vi "Recognize Goal.vi"(5 "Camera Type":T1=enum."MS HD3000 square", 6 "HSV":T5, 7 "Min Score Threshold":i32=70, 8 "Image Dst":T4, 9 "Image In":T4) -> (0 "Highest Average Score":dbl, 1 "Target With Highest Average Score":T2, 2 "All Targets Found":T3(array[cluster]) {"Normalized Rect"."Numeric 5" format="%#_2g"; "Normalized Rect"."Numeric 3" format="%#_2g"; "Normalized Rect"."Numeric 2" format="%#_2g"; "Normalized Rect"."Numeric" format="%#_2g"})   [LabVIEW 2015]
doc: "Performs target recognition on the image passed in. Returns all targets found. Each target includes distance in feet, center X/Y coordinates, and bounding rect coordinates (all coordinates are norminalized from -1 to 1). Also separately returns the target with the highest average score (i.e. most likely to be a real target)."
uses:
  <vilib>/vision/Image Controls.llb/IMAQ Image.ctl
  Camera Types.ctl
  <vilib>/vision/NI_Vision_Development_Module.lvlib
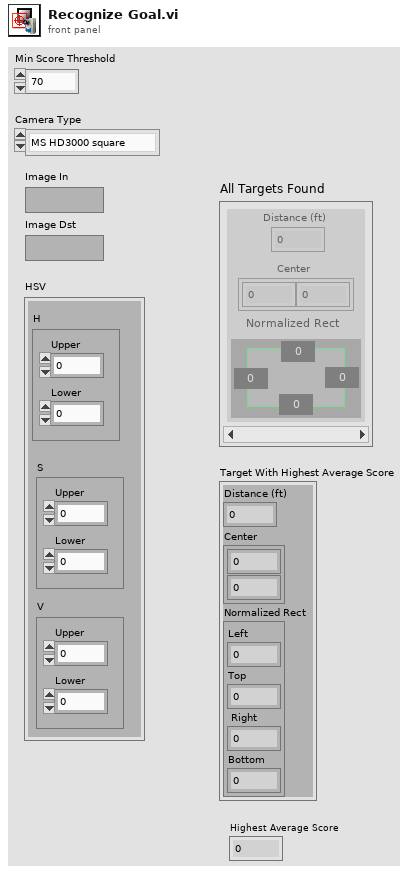
[diagram p1: front panel]
types:
  T1 = typedef "Camera Types.ctl" = enum16{"206", "1011", "1013", "MS HD3000 square", "MS HD3000 640x480"}
  T2 = cluster{"Distance (ft)":dbl, "Center":cluster{dbl, dbl}, "Normalized Rect":cluster{"Left":dbl, "Top":dbl, " Right":dbl, "Bottom":dbl}}
  T3 = cluster{"Distance (ft)":dbl, "Center":cluster{dbl, dbl}, "Normalized Rect":cluster{"Numeric":dbl, "Numeric 2":dbl, "Numeric 3":dbl, "Numeric 5":dbl}}[]
  T4 = typedef "IMAQ Image.ctl" = refnum<image>
  T5 = cluster{"H":cluster{"Upper":dbl, "Lower":dbl}, "S":cluster{"Upper":dbl, "Lower":dbl}, "V":cluster{"Upper":dbl, "Lower":dbl}}
  T6 = typedef "Particle Parameters" = i32
  T7 = cluster{"Bounding box":cluster{"left":dbl, "top":dbl, "right":dbl, "bottom":dbl}, "Aspect Ratio":dbl, "Area to CH":dbl, "X Mask":dbl, "Y Mask":dbl, "Moment":dbl}[]
  T8 = cluster{"Distance (ft)":dbl, "Center":cluster{dbl, dbl}, "Normalized Rect":cluster{"Numeric":dbl, "Numeric 2":dbl, "Numeric 3":dbl, "Numeric 5":dbl}}
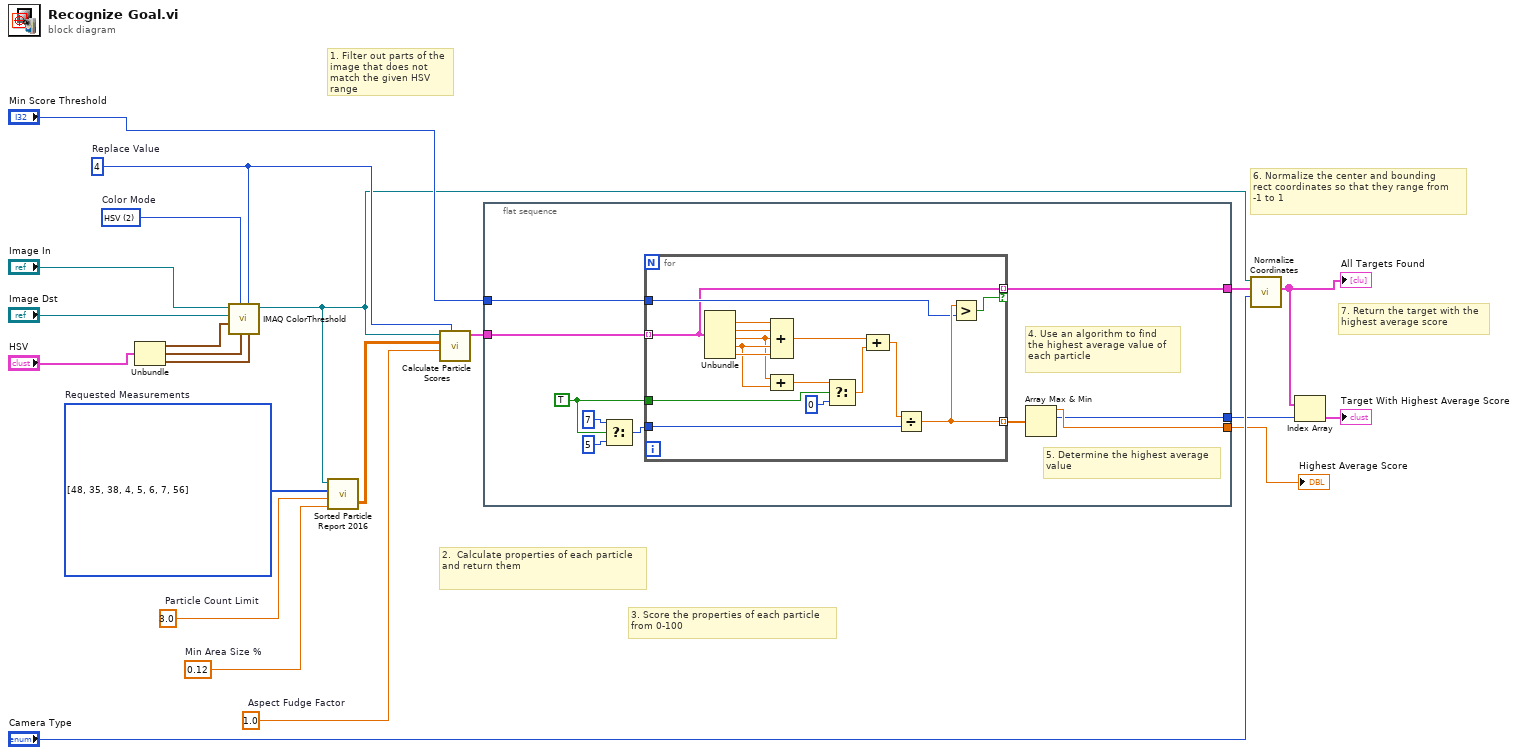
[diagram p0: block diagram]
diagram:
  w11 = 1.0  # Aspect Fudge Factor
  w12 = T6[] [48, 35, 38, 4, 5, 6, 7, 56] items=["Center of Mass X", "Center of Mass Y", "First Pixel X", "First Pixel Y", "Bounding Rect Left", "Bounding Rect Top", "Bounding Rect Right", "Bounding Rect Bottom", "Max Feret Diameter Start X", "Max Feret Diameter Start Y", "Max Feret Diameter End X", "Max Feret Diameter End Y", "Max Horiz. Segment Length Left", "Max Horiz. Segment Length Right", "Max Horiz. Segment Length Row", "-", "Bounding Rect Width", "Bounding Rect Height", "Bounding Rect Diagonal", "Perimeter", "Convex Hull Perimeter", "Holes' Perimeter", "Max Feret Diameter", "Equivalent Ellipse Major Axis", "Equivalent Ellipse Minor Axis", "Equivalent Ellipse Minor Axis (Feret)", "Equivalent Rect Long Side", "Equivalent Rect Short Side", "Equivalent Rect Diagonal", "Equivalent Rect Short Side (Feret)", "Average Horiz. Segment Length", "Average Vert. Segment Length", "Hydraulic Radius", "Waddel Disk Diameter", "-", "Area", "Holes' Area", "Particle & Holes' Area", "Convex Hull Area", "Image Area", "-", "Number of Holes", "Number of Horiz. Segments", "Number of Vert. Segments", "-", "Orientation", "Max Feret Diameter Orientation", "-", "% Area/Image Area", "% Area/(Particle & Holes' Area)", "Ratio of Equivalent Ellipse Axes", "Ratio of Equivalent Rect Sides", "-", "Elongation Factor", "Compactness Factor", "Heywood Circularity Factor", "Type Factor", "-", "Sum X", "Sum Y", "Sum XX", "Sum XY", "Sum YY", "Sum XXX", "Sum XXY", "Sum XYY", "Sum YYY", "-", "Moment of Inertia XX", "Moment of Inertia XY", "Moment of Inertia YY", "Moment of Inertia XXX", "Moment of Inertia XXY", "Moment of Inertia XYY", "Moment of Inertia YYY", "Norm. Moment of Inertia XX", "Norm. Moment of Inertia XY", "Norm. Moment of Inertia YY", "Norm. Moment of Inertia XXX", "Norm. Moment of Inertia XXY", "Norm. Moment of Inertia XYY", "Norm. Moment of Inertia YYY", "Hu Moment 1", "Hu Moment 2", "Hu Moment 3", "Hu Moment 4", "Hu Moment 5", "Hu Moment 6", "Hu Moment 7"]  # Requested Measurements
  w14 = 3.0  # Particle Count Limit
  w15 = 0.12  # Min Area Size %
  w8 = 4  # Replace Value
  w16 = u16 2 items=["RGB", "HSL", "HSV", "HSI"]  # Color Mode
  # "6. Normalize the center and bounding \nrect coordinates so that they range from\n-1 to 1"
  # "7. Return the target with the\nhighest average score"
  # "3. Score the properties of each particle \nfrom 0-100"
  # "2.  Calculate properties of each particle and return them"
  # "1. Filter out parts of the image that does not match the given HSV range"
  n1 = Unbundle("HSV") -> ("H"=w19:cluster{"Upper":dbl, "Lower":dbl}, "S"=w18:cluster{"Upper":dbl, "Lower":dbl}, "V"=w17:cluster{"Upper":dbl, "Lower":dbl})
  n2 = call "IMAQ ColorThreshold"("Blue or Luma or Val or Inten Range"=w17, "Replace Value"=w8, "Green or Sat Range"=w18, "Color Mode"=w16, "Red or Hue Range"=w19, "Image Dst"="Image Dst", "Image Src"="Image In") -> ("Image Dst Out"=w4:T4)  [unwired: 3 in, 1 out]
  n3 = call "Sorted Particle Report 2016.vi"("Min Area Size %"=w15, "Particle Count Limit"=w14, "Pixel Measurements"=w12, "Image in"=w4) -> ("Sorted Data"=w13:dbl[][])  [unwired: 1 out]
  n4 = call "Calculate Particle Scores.vi"("Pixel Value"=w8, "Aspect Fudge Factor"=w11, "Sorted Data"=w13, "Image in"=w4) -> ("Scores"=w10:T7)  [unwired: 7 in]
  n5 = flat-sequence {
    tunnel: w10 -> [w32]
    tunnel: "Min Score Threshold" -> [w31]
    tunnel: [w25] -> w5
    tunnel: [w24] -> w2
    tunnel: [w23] -> w1
    frame #0 {
      w27 = TRUE ("Emphasize Limit Tests")
      # "5. Determine the highest average\nvalue"
      # "4. Use an algorithm to find\nthe highest average value of \neach particle"
      n6 = Select(t=7, s=w27, f=5) -> (s? t:f=w28:i32)
      n7 = for {
        tunnel: w32 -> [w33] mode=indexing
        tunnel: [w33] -> w25 mode=indexing if=w46
        tunnel: [w45] -> w26 mode=indexing
        tunnel: w31 -> [w44]
        tunnel: w27 -> [w37]
        tunnel: w28 -> [w34]
        n8 = Unbundle(w33) -> ("Aspect Ratio"=w48:dbl, "Area to CH"=w47:dbl, "X Mask"=w39:dbl, "Y Mask"=w40:dbl, "Moment"=w41:dbl)  [unwired: 1 out]
        n9 = Compound Arithmetic op=ADD(w48, w47, w39, w40, w41) -> (w43:dbl)
        n10 = Compound Arithmetic op=ADD(w39, w40) -> (w38:dbl)
        n11 = Select(t=w38, s=w37, f=0) -> (s? t:f=w36:dbl)
        n12 = Compound Arithmetic op=ADD(w43, w36) -> (w42:dbl)
        n13 = Divide(x=w42, y=w34) -> (x/y=w45:dbl)
        n14 = Greater?(x=w45, y=w44) -> (0:w46:bool)
      }
      n15 = Array Max & Min(array=w26) -> (max value=w24:dbl, max index (indices)=w23:i32)  [unwired: 2 out]
    }
  }
  n16 = call "Normalize Coordinates.vi"("Camera Type"="Camera Type", "Targets"=w5, "Image in"=w4) -> ("Found Targets"=w7:T3)  [unwired: 7 in, 1 out]
  "All Targets Found" <- w7
  n17 = Index Array(array=w7, index=w1) -> (element=→"Target With Highest Average Score":T8)
  "Highest Average Score" <- w2
